vi "Scalar JSON text to Variant (not inlined).vi"(6 "Type":T1, 8 "error in (no error)":errorcluster, 9 "Variant (Data Type)":variant, 10 "Offset (no whitespace)":i32, 11 "JSON":string) -> (0 "error out":errorcluster, 1 "Variant out":variant)   [LabVIEW 2024, in "JSONtext.lvlib"]
uses:
  JSONtext.lvlib
  Data Type.ctl
  Get String.vi
  Get DBL.vi
  Get Timestamp.vi
  Get I8.vi
  Get I16.vi
  Get I32.vi
  Get I64.vi
  Get U8.vi
  Get U16.vi
  Get U32.vi
  Get U64.vi
  Get Boolean.vi
  Coerce I32 to Variant Intger.vi
  Format Error.vi
  Get SGL.vi
  Advance past String.vi
  String Subset.vi
  Strip Quotes and Unescape.vi
  Get Number Text.vi
  Advance past whitespace.vi
  NaN or null to Integer ERROR.vi
  Advance past Number.vi
  Unescape JSON string.vi
  Advance past Line Ending.vi
  Error Cluster From Error Code.vi
  Parsing Error in converting to LabVIEW type.vi
  JSON type.vi
  Get Refnum Information.vi
  Error Cluster From Code.vi
  Text to Timestamp.vi
  Get Numeric Information.vi
  Get Type Information.vi
  NI_Data Type.lvlib
panel:
  # "NOT INLINED"
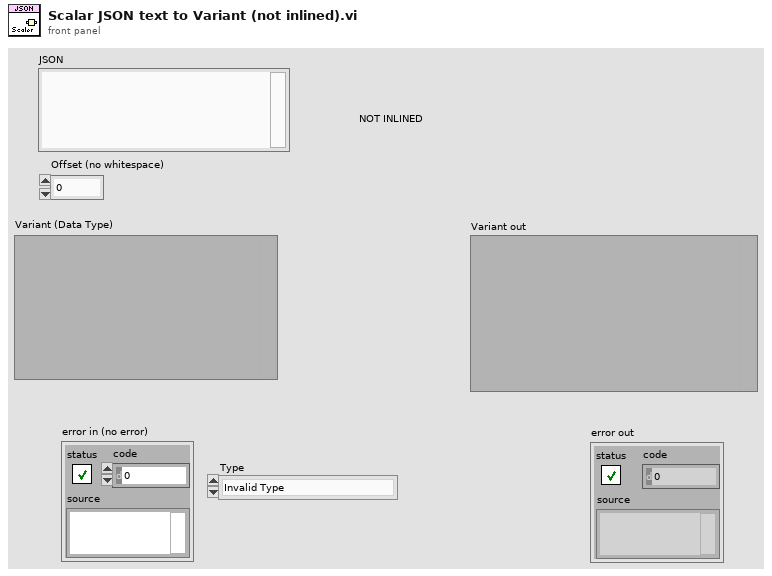
[diagram p1: front panel]
types:
  T1 = typedef "NI_Data Type.lvlib/Data Type.ctl" = enum8{"Invalid Type", "Void", "I8", "I16", "I32", "I64", "U8", "U16", "U32", "U64", "Single Float", "Double Float", "Extended Float", "Single Complex", "Double Complex", "Extended Complex", "Enum U8", "Enum U16", "Enum U32", "Enum U64", "Single Float With Unit", "Double Float With Unit", "Extended Float With Unit", "Single Complex with Unit", "Double Complex with Unit", "Extended Complex with Unit", "Boolean", "String", "Path", "Picture", "Tag", "Array", "Cluster", "Variant", "LV Variant", "Waveform", "Timestamp", "Digital Waveform", "Digital Data", "ExpressData", "Refnum", "External Data", "VI", "Poly VI", "LabVIEW Class Instance", "Fixed Point", "Set Collection", "Map Collection"}
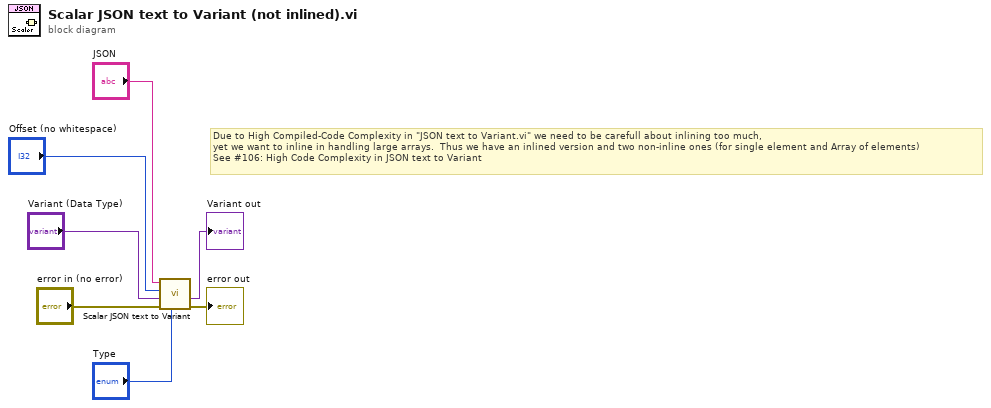
[diagram p0: block diagram]
diagram:
  # "Due to High Compiled-Code Complexity in \"JSON text to Variant.vi\" we need to be carefull about inlining too much,\nyet we want to inline in handling large arrays.  Thus we have an inlined version and two non-inline ones (for single element and Array of elements)\nSee #106: High Code Complexity in JSON text to Variant"
  n1 = call "Scalar JSON text to Variant.vi"("Type"="Type", "error in (no error)"="error in (no error)", "Variant (Data Type)"="Variant (Data Type)", "Offset (no whitespace)"="Offset (no whitespace)", "JSON"="JSON") -> ("error out"=→"error out":errorcluster, "Variant out"=→"Variant out":variant)  [unwired: 5 in]
